vi "Pressure-Main.vi"(8 "error in":errorcluster) -> (0 "error out":errorcluster)   [LabVIEW 2021]
doc: "Use this template to build a simple state machine design pattern. Each state executes code and determines which state to transition to."
uses:
  Controls/Pressure-Data.ctl
  Sensor-Class/Pressure-Transducer_class/Pressure-Transducer.lvclass
  Controls/Pressure-State.ctl
  Pressure Module.lvlib
panel:
  out "output array":u16[](array[numeric])
  out "Pressure":dbl[](array[numeric])
  out "Pressure 2":bool
  out "Status":string
  in  "Read Pressure":bool
  in  "Exit":bool
  # "P1"
  # "Flow 1"
  # "mA    Flow meter"
  # "Flow 2"
  # "mA  Flow meter"
  # "Top"
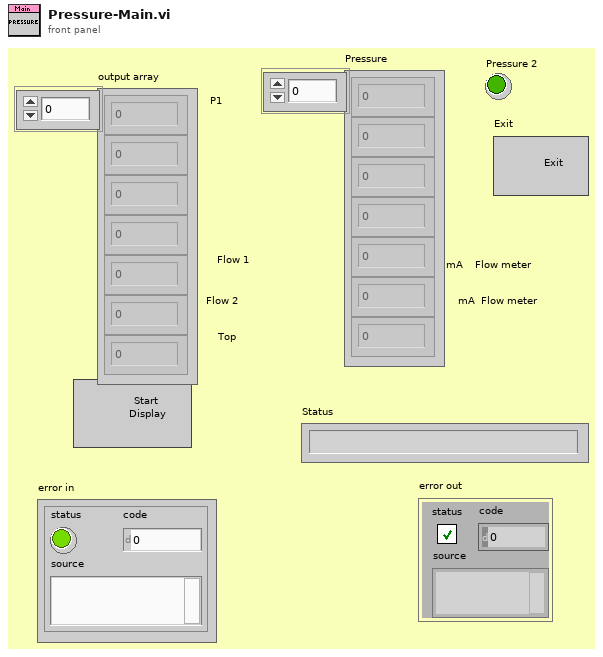
[diagram p1: front panel]
types:
  T1 = typedef "Pressure-State.ctl" = enum16{"Initialize", "Wait for Event", "Data: Pressure", "Data: Pressure-Sym", "Data: Display", "Data: Close", "Error", "Exit"}
  T2 = typedef "Pressure-Data.ctl" = cluster{"?":bool, "Status":string, "Pressure":dbl[], "Modbus-Instr":refnum<class "Pressure-Transducer.lvclass">}
  T3 = typedef "Pressure Module.lvlib/Request Events--cluster.ctl" = cluster{"Stop":refnum<user-event>, "Start Display Pressure":refnum<user-event>}
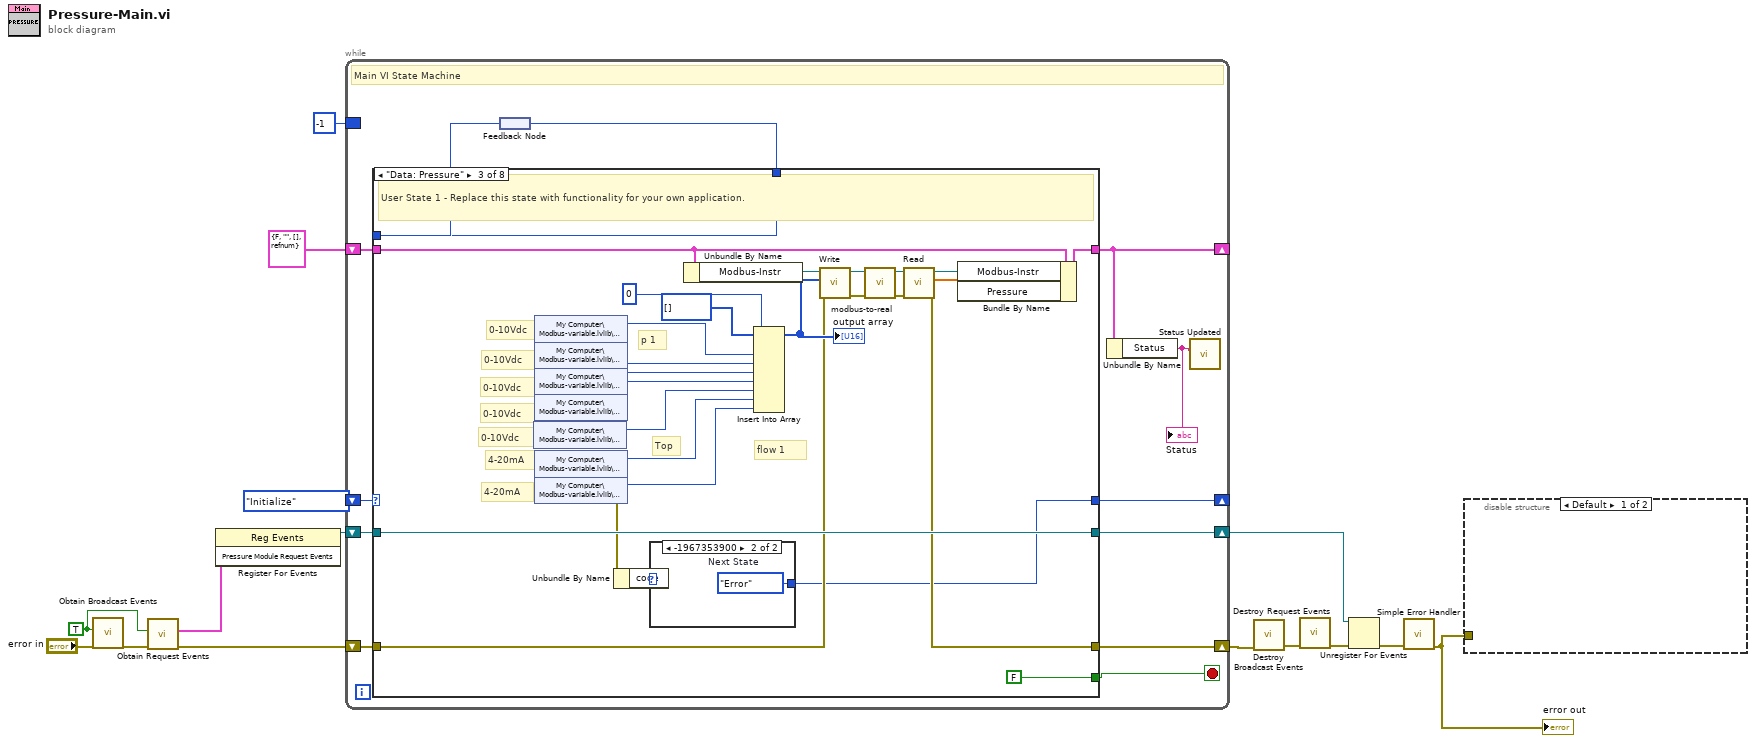
[diagram p0: block diagram]
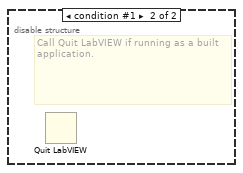
[diagram p2: hidden frame]
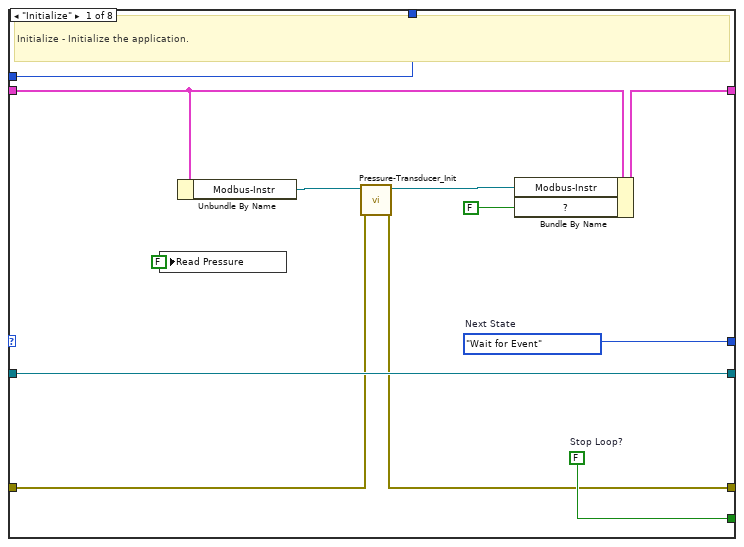
[diagram p3: hidden frame]
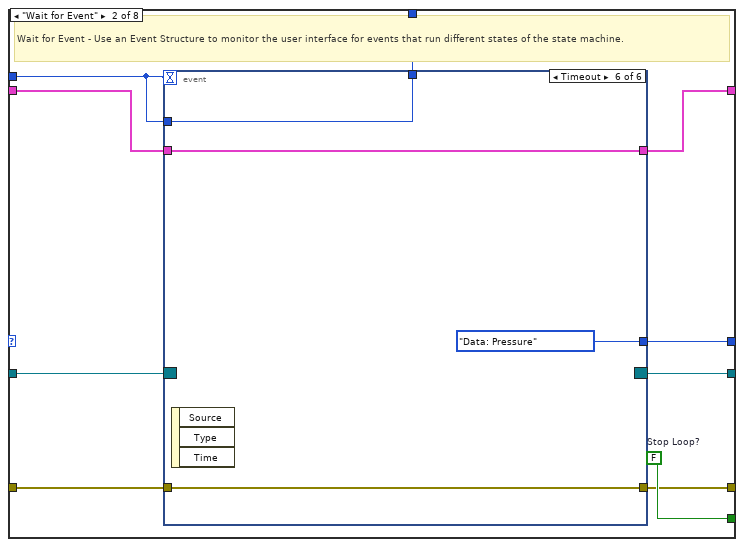
[diagram p4: hidden frame]
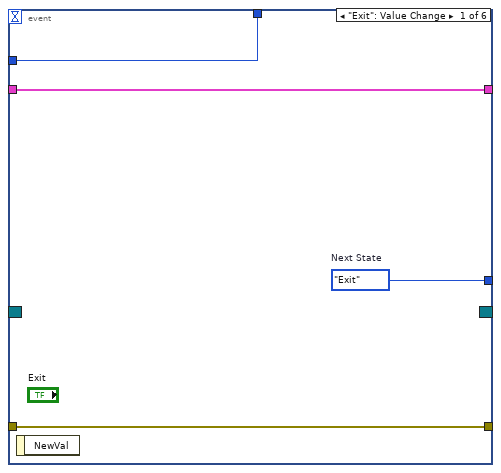
[diagram p5: hidden frame]
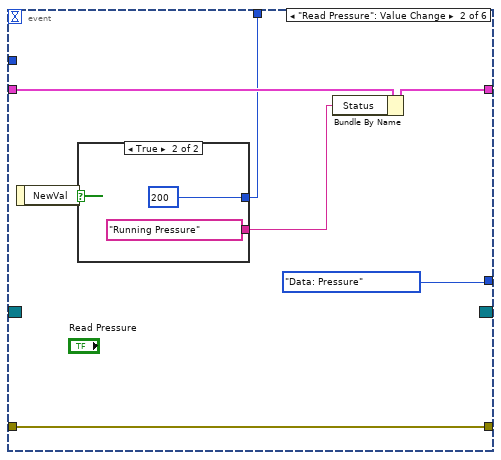
[diagram p6: hidden frame]
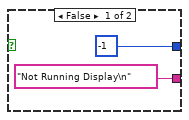
[diagram p7: hidden frame]
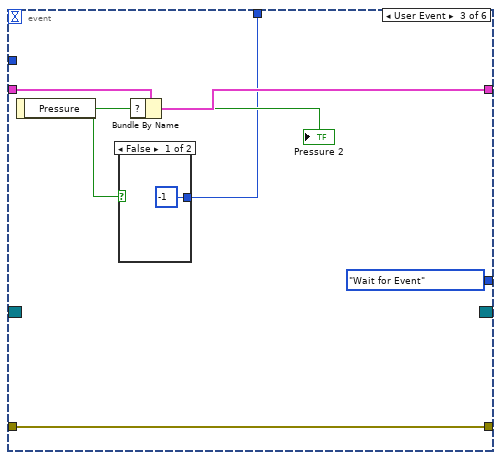
[diagram p8: hidden frame]
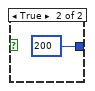
[diagram p9: hidden frame]
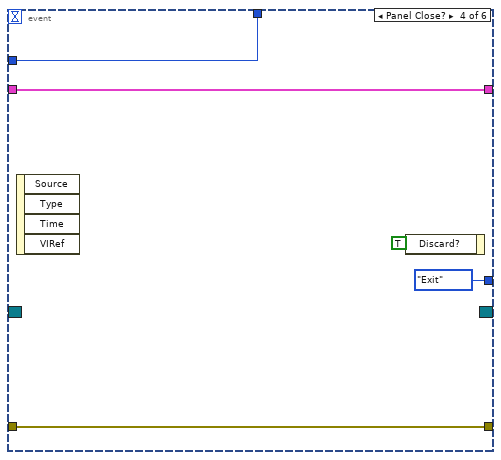
[diagram p10: hidden frame]
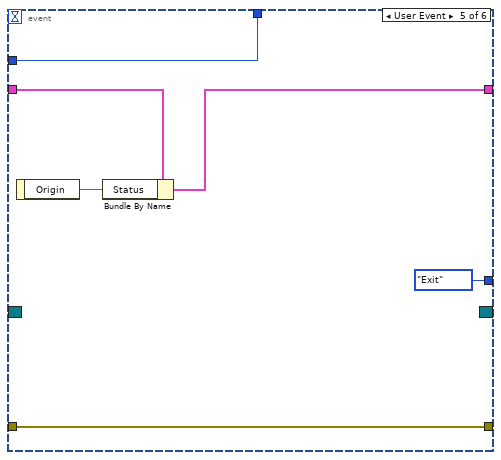
[diagram p11: hidden frame]
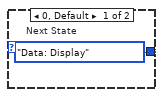
[diagram p12: hidden frame]
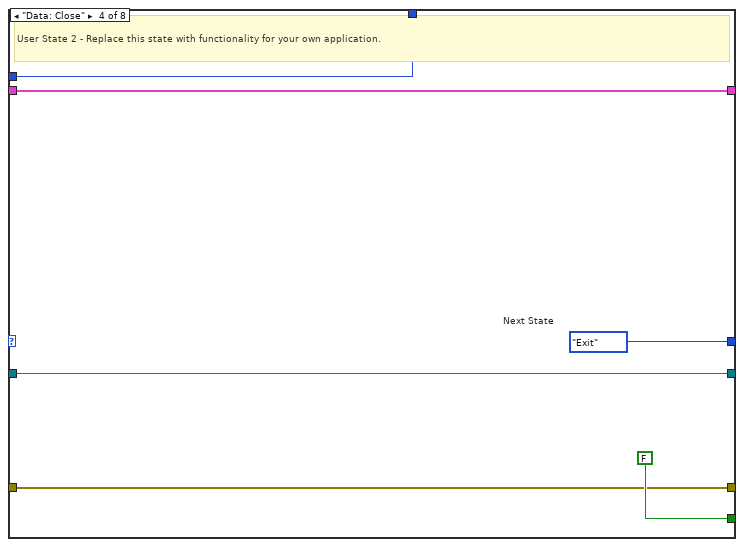
[diagram p13: hidden frame]
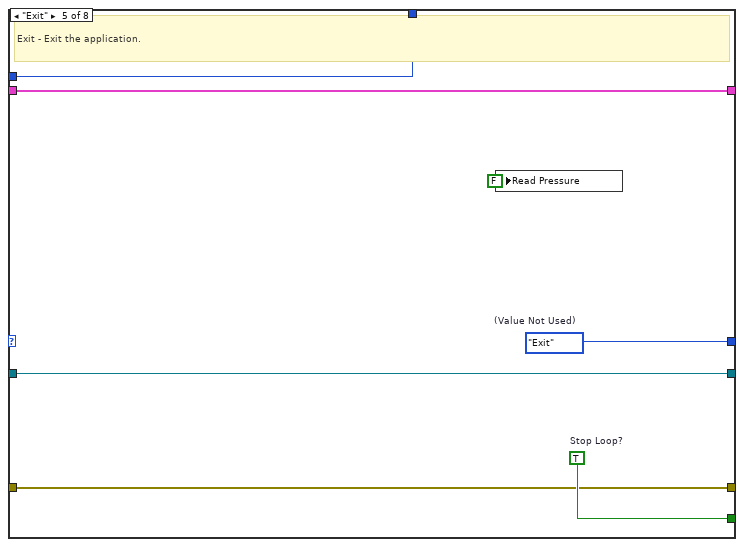
[diagram p14: hidden frame]
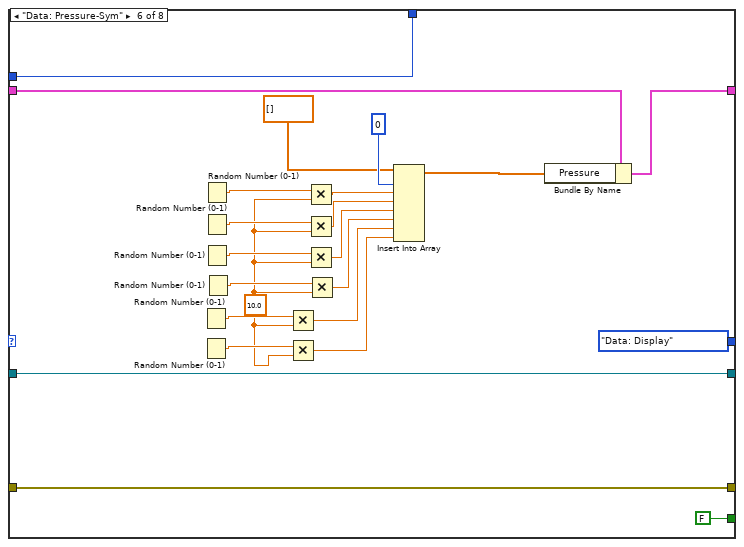
[diagram p15: hidden frame]
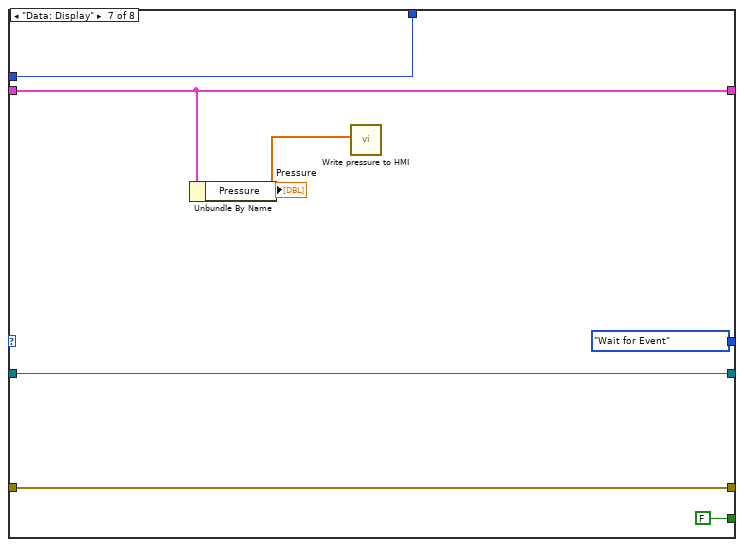
[diagram p16: hidden frame]
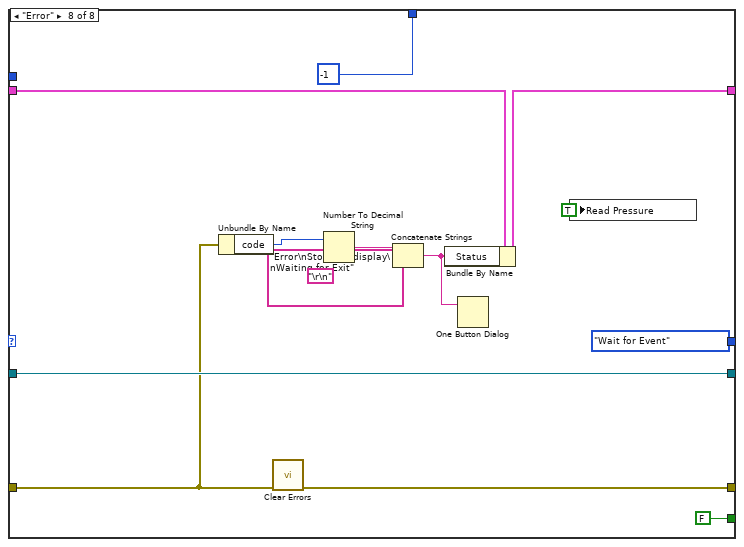
[diagram p17: hidden frame]
diagram:
  w10 = TRUE ("Create New?")
  n1 = call "Obtain Broadcast Events.vi"("error in (no error)"="error in", "Create New?"=w10) -> ("error out"=w13:errorcluster)  [unwired: 8 in, 1 out]
  n2 = call "Obtain Request Events.vi"("error in (no error)"=w13, "Create New?"=w10) -> ("error out"=w11:errorcluster, "Pressure Module Request Events"=w9:T3)  [unwired: 8 in]
  n3 = register-events(w9) -> (reference out=w8:refnum<event-registration>)  [unwired: 2 in, 1 out]
  n4 = while {
    shift-right: [w26] -> _
    shift-left: Pressure-State."Initialize" ("States") -> [w27]
    shift-right: [w19] -> _
    shift-left: T2 {"?"=FALSE, "Status"="", "Pressure"=[], "Modbus-Instr"=refnum} ("Data") -> [w25]
    shift-right: [w22] -> w5
    shift-left: w11 -> [w24]
    shift-right: [w21] -> w3
    shift-left: w8 -> [w20]
    border: -1 -> [_]
    stop <- w23 stop-if-true
    # "Main VI State Machine"
    n5 = feedback #1() -> (w17:i32)
    n6 = case shown="\"Data: Pressure\"" w27 {
      tunnel: [w39 w49 w93 w122 w129 Pressure-State."Data: Display" ("(Value Not Used)") Pressure-State."Wait for Event" ("(Value Not Used)") Pressure-State."Wait for Event" ("(Value Not Used)")] -> w26
      tunnel: [w38 w48 FALSE ("Stop Loop?") FALSE ("Stop Loop?") w127 FALSE ("Stop Loop?") FALSE ("Stop Loop?") FALSE ("Stop Loop?")] -> w23
      tunnel: w25 -> [w34 w47 w98 w120 w128 w136 w157 w171]
      tunnel: [w37 w46 w97 w120 w128 w135 w157 w170] -> w19
      tunnel: w24 -> [w31 w45 w100 w119 w126 w152 w159 w172]
      tunnel: [w30 w44 w99 w119 w126 w152 w159 w167] -> w22
      tunnel: [w35 w43 w113 w118 w125 w151 w158 w173] -> w21
      tunnel: w20 -> [w35 w42 w113 w118 w125 w151 w158 w173]
      tunnel: w17 -> [w29 w41 w92 w117 w124 w130 w153 _]
      tunnel: [w29 w40 w92 w117 w124 w130 w153 -1] -> w16
      frame "Initialize" {
        w38 = FALSE  # Stop Loop?
        w39 = Pressure-State."Wait for Event"  # Next State
        # "Initialize - Initialize the application."
        n7 = local write "Read Pressure"(FALSE ("Read Pressure")) -> ()
        n8 = Unbundle By Name(w34) -> ("Modbus-Instr"=w33:refnum<class "Pressure-Transducer.lvclass">)
        n9 = call "Pressure-Transducer_Init.vi"("error in (no error)"=w31, "object in"=w33) -> ("error out"=w30:errorcluster, "object out"=w32:refnum<class "Pressure-Transducer.lvclass">)  [unwired: 8 in]
        n10 = Bundle By Name(cluster=w34, "Modbus-Instr"=w32, "?"=FALSE ("Replace_Me_Boolean")) -> (w37:T2)
      }
      frame "Wait for Event" {
        w48 = FALSE  # Stop Loop?
        # "Wait for Event - Use an Event Structure to monitor the user interface for events that run different states of the state machine."
        n11 = event shown="[5] Timeout" {
          selector: w42 -> [_ _ _ _ _ _]
          dyn-events: [_ _ _ _ _ _] -> w43
          timeout: w41 -> [_ _ _ _ _ _]
          tunnel: [w53 Pressure-State."Data: Pressure" ("States") Pressure-State."Wait for Event" ("Initial State") Pressure-State."Exit" ("Initial State") Pressure-State."Exit" ("Initial State") Pressure-State."Data: Pressure" ("Initial State")] -> w49
          tunnel: w47 -> [w52 w60 w69 w77 w81 w86]
          tunnel: [w52 w59 w68 w77 w80 w86] -> w46
          tunnel: w45 -> [w51 w58 w70 w76 w83 w87]
          tunnel: [w51 w58 w70 w76 w83 w87] -> w44
          tunnel: w41 -> [w50 _ _ w73 w78 w84]
          tunnel: [w50 w55 w65 w73 w78 w84] -> w40
          event "Exit": Value Change {
            w53 = Pressure-State."Exit"  # Next State
            n12 = event-data() -> ()  [unwired: 1 in, 1 out]
          }
          event "Read Pressure": Value Change {
            n13 = event-data() -> ("NewVal"=w56:bool)  [unwired: 1 in]
            n14 = case shown="True" w56 {
              tunnel: [-1 200] -> w55
              tunnel: ["Not Running Display\n" ("Running User State 1") "Running Pressure" ("Running User State 1")] -> w54
              frame False {
              }
              frame True {
              }
            }
            n15 = Bundle By Name(cluster=w60, "Status"=w54) -> (w59:T2)
          }
          event User Event {
            n16 = event-data() -> ("Pressure"=w66:bool)  [unwired: 1 in]
            "Pressure 2" <- w66
            n17 = case shown="False" w66 {
              tunnel: [-1 200] -> w65
              frame False {
              }
              frame True {
              }
            }
            n18 = Bundle By Name(cluster=w69, "?"=w66) -> (w68:T2)
          }
          event Panel Close? {
            n19 = event-data() -> ()  [unwired: 1 in, 4 out]
            n20 = event-data("Discard?"=TRUE) -> ()  [unwired: 1 in, 1 out]
          }
          event User Event {
            n21 = event-data() -> ("Origin"=w79:string)  [unwired: 1 in]
            n22 = Bundle By Name(cluster=w81, "Status"=w79) -> (w80:T2)
          }
          event Timeout {
            n23 = event-data() -> ()  [unwired: 1 in, 3 out]
          }
        }
      }
      frame "Data: Pressure" {
        # "Top"
        # "flow 1"
        # "p 1"
        # "4-20mA"
        # "0-10Vdc"
        # "0-10Vdc"
        # "0-10Vdc"
        # "0-10Vdc"
        # "0-10Vdc"
        # "4-20mA"
        # "User State 1 - Replace this state with functionality for your own application."
        n24 = shared-variable "My Computer\\Modbus-variable.lvlib\\400023"() -> (w91:u16)  [unwired: 1 in, 1 out]
        n25 = shared-variable "My Computer\\Modbus-variable.lvlib\\400017"() -> (w111:u16)  [unwired: 1 in, 1 out]
        n26 = shared-variable "My Computer\\Modbus-variable.lvlib\\400018"() -> (w109:u16)  [unwired: 1 in, 1 out]
        n27 = shared-variable "My Computer\\Modbus-variable.lvlib\\400019"() -> (w108:u16)  [unwired: 1 in, 1 out]
        n28 = shared-variable "My Computer\\Modbus-variable.lvlib\\400020"() -> (w107:u16)  [unwired: 1 in, 1 out]
        n29 = shared-variable "My Computer\\Modbus-variable.lvlib\\400021"() -> (w90:u16)  [unwired: 1 in, 1 out]
        n30 = shared-variable "My Computer\\Modbus-variable.lvlib\\400022"() -> (w89:u16, error out=w88:errorcluster)  [unwired: 1 in]
        n31 = Unbundle By Name(w88) -> ("code"=w94:i32)
        n32 = case shown="-1967353900" w94 {
          tunnel: [w115 w116] -> w93
          frame 0, Default {
            w115 = Pressure-State."Data: Display"  # Next State
          }
          frame -1967353900 {
            w116 = Pressure-State."Error"  # Next State
          }
        }
        n33 = Unbundle By Name(w98) -> ("Modbus-Instr"=w102:refnum<class "Pressure-Transducer.lvclass">)
        n34 = Insert Into Array(array=u16[] [], index=0, new element #1=w111, new element #2=w109, new element #3=w108, new element #4=w107, new element #5=w91, new element #6=w90, new element #7=w89) -> (w101:u16[])
        "output array" <- w101
        n35 = call-dynamic "Write.vi"("error in (no error)"=w100, "Modbus-Reg"=w101, "object in"=w102) -> ("error out"=w105:errorcluster, "object out"=w106:refnum<class "Pressure-Transducer.lvclass">)  [unwired: 7 in]
        n36 = call-dynamic "modbus-to-real.vi"("error in (no error)"=w105, "object in"=w106) -> ("error out"=w103:errorcluster, "object out"=w104:refnum<class "Pressure-Transducer.lvclass">)  [unwired: 8 in]
        n37 = call-dynamic "Read.vi"("error in (no error)"=w103, "object in"=w104) -> ("error out"=w99:errorcluster, "Data"=w95:dbl[], "object out"=w96:refnum<class "Pressure-Transducer.lvclass">)  [unwired: 7 in]
        n38 = Bundle By Name(cluster=w98, "Modbus-Instr"=w96, "Pressure"=w95) -> (w97:T2)
      }
      frame "Data: Close" {
        w122 = Pressure-State."Exit"  # Next State
        # "User State 2 - Replace this state with functionality for your own application."
      }
      frame "Exit" {
        w127 = TRUE  # Stop Loop?
        w129 = Pressure-State."Exit"  # (Value Not Used)
        # "Exit - Exit the application."
        n39 = local write "Read Pressure"(FALSE ("Read Pressure")) -> ()
      }
      frame "Data: Pressure-Sym" {
        w144 = 10.0 ("y")
        n40 = Random Number (0-1)() -> (number: 0 to 1=w146:dbl)
        n41 = Random Number (0-1)() -> (number: 0 to 1=w145:dbl)
        n42 = Random Number (0-1)() -> (number: 0 to 1=w150:dbl)
        n43 = Random Number (0-1)() -> (number: 0 to 1=w149:dbl)
        n44 = Random Number (0-1)() -> (number: 0 to 1=w148:dbl)
        n45 = Random Number (0-1)() -> (number: 0 to 1=w147:dbl)
        n46 = Multiply(x=w146, y=w144) -> (x*y=w138:dbl)
        n47 = Multiply(x=w145, y=w144) -> (x*y=w137:dbl)
        n48 = Multiply(x=w150, y=w144) -> (x*y=w142:dbl)
        n49 = Multiply(x=w149, y=w144) -> (x*y=w141:dbl)
        n50 = Multiply(x=w148, y=w144) -> (x*y=w140:dbl)
        n51 = Multiply(x=w147, y=w144) -> (x*y=w139:dbl)
        n52 = Insert Into Array(array=dbl[] [], index=0, new element #1=w142, new element #2=w141, new element #3=w140, new element #4=w139, new element #5=w138, new element #6=w137) -> (w134:dbl[])
        n53 = Bundle By Name(cluster=w136, "Pressure"=w134) -> (w135:T2)
      }
      frame "Data: Display" {
        n54 = Unbundle By Name(w157) -> ("Pressure"=w154:dbl[])
        "Pressure" <- w154
        n55 = call "Write pressure to HMI.vi"("Pressure"=w154) -> ()  [unwired: 10 in, 1 out]
      }
      frame "Error" {
        n56 = Unbundle By Name(w172) -> ("code"=w165:i32)
        n57 = call <vilib>:"Clear Errors.vi"("error in (no error)"=w172) -> ("error out"=w167:errorcluster)  [unwired: 5 in, 1 out]
        n58 = Number To Decimal String(number=w165) -> (decimal integer string=w164:string)  [unwired: 1 in]
        n59 = Concatenate Strings(w164, "\r\n", "Error\nStopping display\nWaiting for Exit" ("string")) -> (w161:string)
        n60 = Bundle By Name(cluster=w171, "Status"=w161) -> (w170:T2)
        n61 = One Button Dialog(message=w161) -> ()  [unwired: 1 in, 1 out]
        n62 = local write "Read Pressure"(TRUE ("Read Pressure")) -> ()
      }
    }
    n63 = feedback-in #1(w16) -> ()
    n64 = Unbundle By Name(w19) -> ("Status"=w18:string)
    "Status" <- w18
    n65 = call "Status Updated.vi"("Status"=w18) -> ()  [unwired: 10 in, 1 out]
  }
  n66 = call "Destroy Broadcast Events.vi"("error in (no error)"=w5) -> ("error out"=w7:errorcluster)  [unwired: 10 in]
  n67 = call "Destroy Request Events.vi"("error in (no error)"=w7) -> ("error out"=w6:errorcluster)  [unwired: 10 in]
  n68 = Unregister For Events(event registration refnum=w3, error in=w6) -> (error out=w4:errorcluster)
  n69 = call <vilib>:"Simple Error Handler.vi"("error in (no error)"=w4) -> ("error out"=w14:errorcluster)  [unwired: 4 in, 4 out]
  "error out" <- w14
  n70 = disable-structure shown="Default" {
    disable-tunnel: w14 -> [_ _]
    frame condition #0 (active) {
    }
    frame condition #1 {
      # "Call Quit LabVIEW if running as a built application."
      n71 = Quit LabVIEW() -> ()  [unwired: 1 in]
    }
  }
